vi "FirePneumatic.vi"   [LabVIEW 2012]
uses:
  State_Machine_Enum.ctl
  <vilib>/Rock Robotics/WPI/Solenoid/WPI_SolenoidValue.ctl
  <vilib>/Rock Robotics/WPI/Solenoid/WPI_SolenoidSetEnum.vi
  Robot Global Data.vi
  <vilib>/Rock Robotics/WPI/Compressor/WPI_CompressorGetSetRefNum.vi
types:
  T1 = typedef "State_Machine_Enum.ctl" = enum16{"Init", "Idle", "Start", "Do", "Stop"}
  T2 = typedef "WPI_SolenoidValue.ctl" = enum16{"Off", "On", "Forward", "Reverse"}
  T3 = typedef "WPI_CompressorDevRef.ctl" = cluster{"DevStatus":errorcluster, "DigitalInputDevRef":T4, "RelayDevRef":T7}
  T4 = typedef "WPI_DigitalInputDevRef.ctl" = cluster{"DevStatus":errorcluster, "DIO Channel":T5, "Digital Module":T6}
  T5 = typedef "FPGA_DIOChannel.ctl" = enum8{"DIO 1", "DIO 2", "DIO 3", "DIO 4", "DIO 5", "DIO 6", "DIO 7", "DIO 8", "DIO 9", "DIO 10", "DIO 11", "DIO 12", "DIO 13", "DIO 14", "Invalid"}
  T6 = typedef "FPGA_TypedefDigitalModule.ctl" = enum16{"Digital Module 1", "Digital Module 2"}
  T7 = typedef "WPI_RelayDevRef.ctl" = cluster{"DevStatus":errorcluster, "Relay Channel":T8, "Digital Module":T6, "Relay Direction":T9}
  T8 = typedef "FPGA_DIORelayChannel.ctl" = enum8{"Relay 1", "Relay 2", "Relay 3", "Relay 4", "Relay 5", "Relay 6", "Relay 7", "Relay 8", "Invalid"}
  T9 = typedef "WPI_RelayDirection.ctl" = enum16{"Both directions", "Forward only", "Reverse only"}
  T10 = typedef "WPI_SolenoidDevRef.ctl" = cluster{"DevStatus":errorcluster, "Solenoid Module":T11, "Forward Solenoid Channel":T12, "Reverse Solenoid Channel":T12}
  T11 = typedef "FPGA_TypedefSolenoidModule.ctl" = enum16{"Solenoid Module 1", "Solenoid Module 2"}
  T12 = typedef "WPI_SolenoidChannel.ctl" = enum8{"Solenoid 1", "Solenoid 2", "Solenoid 3", "Solenoid 4", "Solenoid 5", "Solenoid 6", "Solenoid 7", "Solenoid 8", "Invalid"}
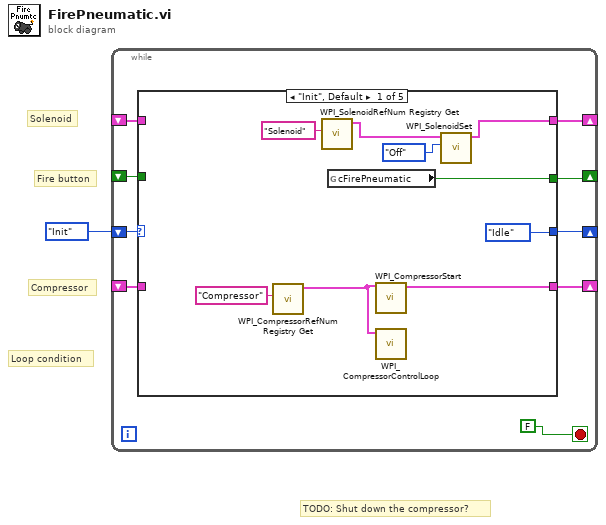
[diagram p0: block diagram]
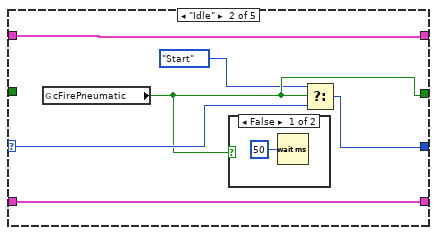
[diagram p2: hidden frame]
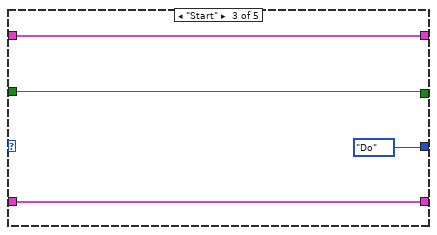
[diagram p4: hidden frame]
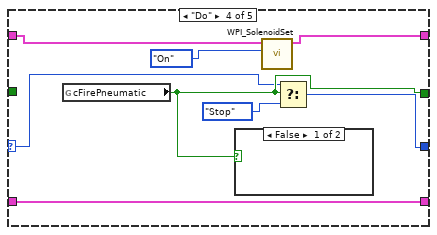
[diagram p5: hidden frame]
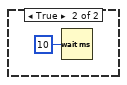
[diagram p6: hidden frame]
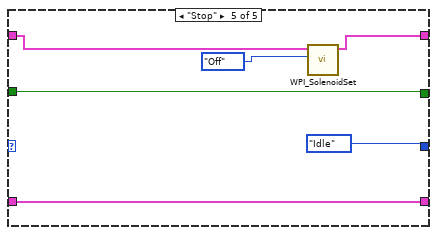
[diagram p7: hidden frame]
diagram:
  # "TODO: Shut down the compressor?"
  # "Loop condition"
  # "Fire button"
  # "Solenoid"
  # "Compressor"
  n1 = while {
    shift-right: [w3] -> _
    shift-left: State_Machine_Enum."Init" ("State") -> [w10]
    shift-right: [w9] -> _
    shift-left: _ -> [w8]
    shift-right: [w7] -> _
    shift-left: _ -> [w6]
    shift-right: [w5] -> _
    shift-left: _ -> [w4]
    stop <- FALSE stop-if-true
    n2 = case shown="\"Init\", Default" w10 {
      selector: w10 -> [_ w24 _ w31 _]
      tunnel: [w17 w25 w28 w34 w41] -> w9
      tunnel: w8 -> [_ w25 w28 w34 w41]
      tunnel: [w11 w20 w30 w36 w43] -> w7
      tunnel: w6 -> [_ w20 w30 w37 w44]
      tunnel: [w15 w22 w29 w33 w42] -> w5
      tunnel: w4 -> [_ _ w29 _ w42]
      tunnel: [State_Machine_Enum."Idle" ("State") w23 State_Machine_Enum."Do" ("State") w35 State_Machine_Enum."Idle" ("State")] -> w3
      frame "Init", Default {
        n3 = call <vilib>:"WPI_CompressorRefNum Registry Get.vi"("refnum name"="Compressor") -> ("CompressorDevRef"=w19:T3)  [unwired: 9 in, 1 out]
        n4 = call <vilib>:"WPI_SolenoidRefNum Registry Get.vi"("refnum name"="Solenoid") -> ("SolenoidDevRef"=w12:T10)  [unwired: 9 in, 1 out]
        n5 = global read "Robot Global Data.vi" "cFirePneumatic"() -> (w15:bool)
        n6 = call <vilib>:"WPI_CompressorStart.vi"("CompressorDevRef"=w19) -> ("CompressorDevRef"=w17:T3)  [unwired: 1 in, 9 out]
        n7 = call <vilib>:"WPI_CompressorControlLoop.vi"("CompressorDevRef"=w19) -> ()  [unwired: 11 in]
        n8 = call-poly <vilib>:"WPI_SolenoidSet.vi"("Value"=WPI_SolenoidValue."Off", "SolenoidDevRef"=w12) -> ("SolenoidDevRef"=w11:T10)  [unwired: 1 in, 8 out]
      }
      frame "Idle" {
        n9 = global read "Robot Global Data.vi" "cFirePneumatic"() -> (w22:bool)
        n10 = case shown="False" w22 {
          frame False {
            n11 = Wait (ms)(milliseconds to wait=u32 50) -> ()  [unwired: 1 out]
          }
          frame True {
          }
        }
        n12 = Select(t=State_Machine_Enum."Start" ("State"), s=w22, f=w24) -> (s? t:f=w23:T1)
      }
      frame "Start" {
      }
      frame "Do" {
        n13 = global read "Robot Global Data.vi" "cFirePneumatic"() -> (w33:bool)
        n14 = case shown="False" w33 {
          frame False {
          }
          frame True {
            n15 = Wait (ms)(milliseconds to wait=u32 10) -> ()  [unwired: 1 out]
          }
        }
        n16 = call-poly <vilib>:"WPI_SolenoidSet.vi"("Value"=WPI_SolenoidValue."On", "SolenoidDevRef"=w37) -> ("SolenoidDevRef"=w36:T10)  [unwired: 1 in, 8 out]
        n17 = Select(t=w31, s=w33, f=State_Machine_Enum."Stop" ("State")) -> (s? t:f=w35:T1)
      }
      frame "Stop" {
        n18 = call-poly <vilib>:"WPI_SolenoidSet.vi"("Value"=WPI_SolenoidValue."Off", "SolenoidDevRef"=w44) -> ("SolenoidDevRef"=w43:T10)  [unwired: 1 in, 8 out]
      }
    }
  }
